vi "SaveImage.vi"(0 "object in":refnum<class "Experiment.lvclass">, 2 "Image":T1, 3 "ImageNumber":i32, 5 "error in (no error)":errorcluster) -> (14 "object out":refnum<class "Experiment.lvclass">, 16 "Imagepath":path, 19 "error out":errorcluster)   [LabVIEW 2019, in "Experiment.lvclass"]
uses:
  Experiment.lvclass
  <vilib>/vision/Image Controls.llb/IMAQ Image.ctl
  Experiment.lvclass/Experiment.ctl
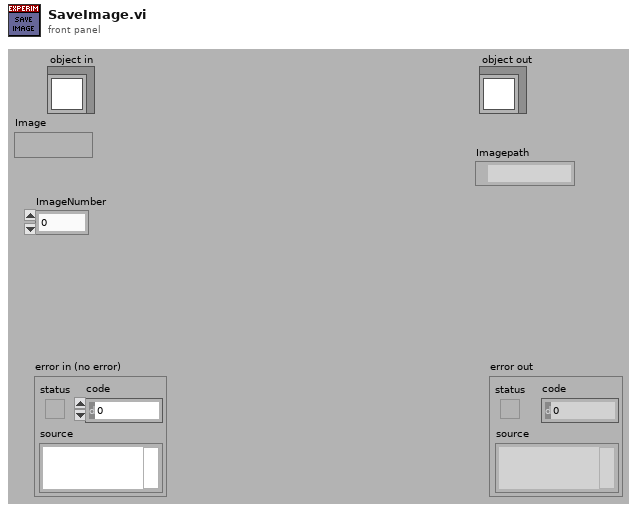
[diagram p1: front panel]
types:
  T1 = typedef "IMAQ Image.ctl" = refnum<image>
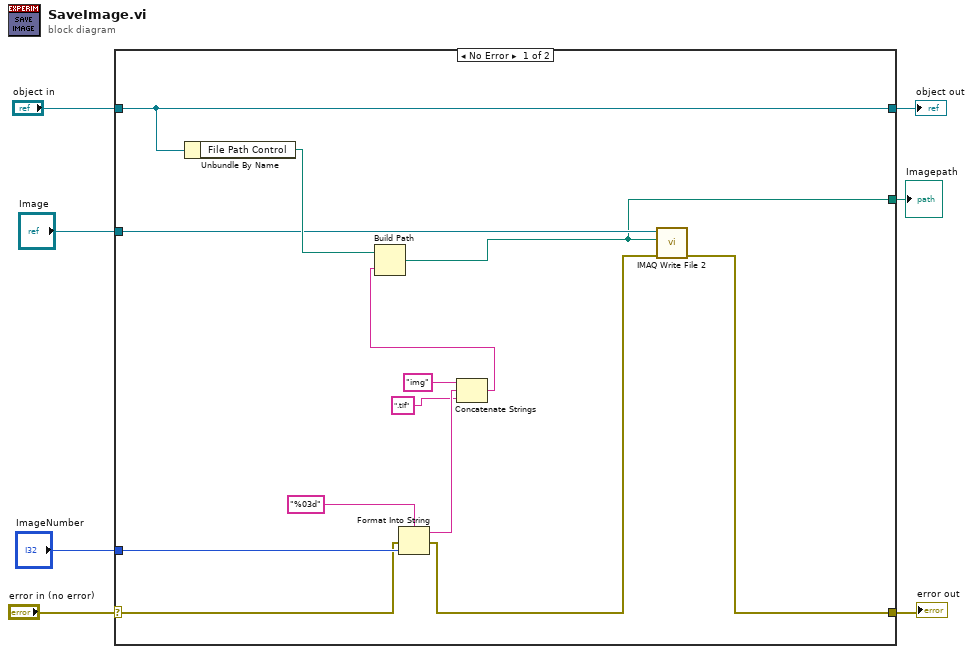
[diagram p0: block diagram]
diagram:
  n1 = case shown="No Error" "error in (no error)" {
    selector: "error in (no error)" -> [w11 w22]
    tunnel: [w12 w22] -> w6
    tunnel: [w20 w21] -> w4
    tunnel: "object in" -> [w20 w21]
    tunnel: "ImageNumber" -> [w17 _]
    tunnel: "Image" -> [w13 _]
    tunnel: [w9 _] -> w1
    frame No Error {
      n2 = Unbundle By Name(w20) -> ("File Path Control"=w19:path)
      n3 = Format Into String(format string="%03d", error in=w11, w17) -> (resulting string=w15:string, error out=w10:errorcluster)  [unwired: 1 in]
      n4 = Concatenate Strings("img" ("string"), w15, ".tif" ("string")) -> (w14:string)
      n5 = Build Path(base path=w19, name or relative path=w14) -> (appended path=w9:path)
      n6 = call-poly "IMAQ Write File 2"("error in (no error)"=w10, "File Path"=w9, "Image"=w13) -> ("error out"=w12:errorcluster)  [unwired: 7 in, 1 out]
    }
    frame Error {
    }
  }
  "error out" <- w6
  "object out" <- w4
  "Imagepath" <- w1
